vi "LabVIEW Coordinates to Picture Coordinates.vi"(8 "错误输入":errorcluster, 10 "控件引用":refnum<vi>, 11 "LabVIEW坐标":cluster{"水平":i32, "垂直":i32}) -> (0 "错误输出":errorcluster, 3 "图片控件坐标":cluster{"水平":i32, "垂直":i32})   [LabVIEW 2012]
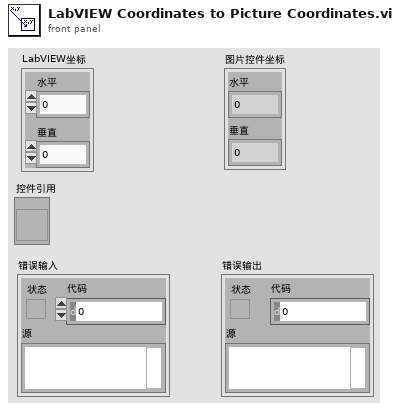
[diagram p1: front panel]
types:
  T1 = typedef "LVBoundsTypeDef.ctl" = cluster{"Width":u32, "Height":u32}
  T2 = typedef "LVPositionTypeDef.ctl" = cluster{"Left":i32, "Top":i32}
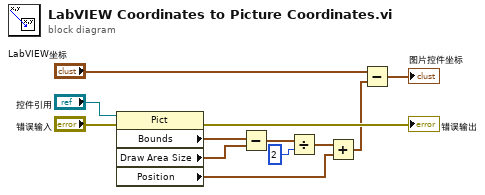
[diagram p0: block diagram]
diagram:
  n1 = property on="属性节点" class="Pict"(reference="控件引用", error in="错误输入") -> (error out=→"错误输出":errorcluster, "Bounds"=w3:T1, "Draw Area Size"=w4:T1, "Position"=w8:T2)  [unwired: 1 out]
  n2 = Subtract ("减")(x=w3, y=w4) -> (x-y=w6:T1)
  n3 = Divide ("除")(x=w6, y=2) -> (x/y=w7:cluster{"Width":dbl, "Height":dbl})
  n4 = Add ("加")(x=w7, y=w8) -> (x+y=w10:cluster{dbl, dbl})
  n5 = Subtract ("减")(x="LabVIEW坐标", y=w10) -> (x-y=→"图片控件坐标":cluster{dbl, dbl})
